vi "SemaphoreResultManager.vi"() -> ()   [LabVIEW 2011]
panel:
  out "ResultManager":cluster{"InstancePtr":u64}
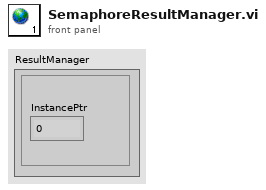
[diagram p1: front panel]
diagram:
